vi "Configure Air High Temperature Limit.vi"(8 "error in (no error)":errorcluster, 9 "Air High Temperature Limit (225)":dbl=225.0 min=25.0 max=225.0 step=1.0, 11 "VISA resource name":refnum<visa-resource-name>) -> (0 "error out":errorcluster, 3 "VISA resource name out":refnum<visa-resource-name>)   [LabVIEW 2010, in "Temptronic TP04300.lvlib"]
doc: "This VI configures air high temperature limit for TP04300 instrument.\n\n<b>Air High Temperature Limit</b> configures the maximum allowable air\ntemperature in Celsius for both air and DUT modes. Out of range error will be generated \nif a setpoint exceeds this value.\n\nDefault Value: 225.0\nValid Range: 25.0 - 225.0"
uses:
  Temptronic TP04300.lvlib
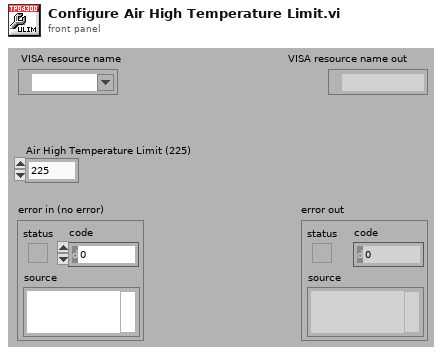
[diagram p1: front panel]
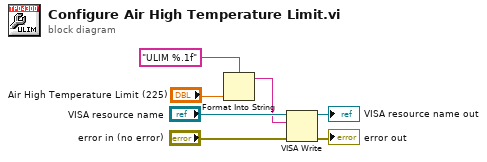
[diagram p0: block diagram]
diagram:
  n1 = Format Into String(format string="ULIM %.1f" ("multi-line string"), "Air High Temperature Limit (225)") -> (resulting string=w3:string)  [unwired: 2 in, 1 out]
  n2 = VISA Write(VISA resource name="VISA resource name", write buffer=w3, error in (no error)="error in (no error)") -> (VISA resource name out=→"VISA resource name out":refnum<visa-resource-name>, error out=→"error out":errorcluster)  [unwired: 1 out]
